vi "Match Terminals.vi"(10 "Terms[]":refnum<vi>[](array[refnum]), 11 "Terminals":T1[](array[typedef])) -> (3 "Terminals Out":T1[](array[typedef]))   [LabVIEW 2025]
uses:
  Controls/Terminal.ctl
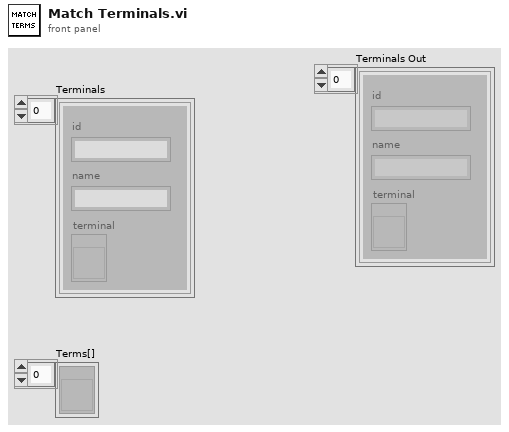
[diagram p1: front panel]
types:
  T1 = typedef "Terminal.ctl" = cluster{"id":string, "name":string, "terminal":refnum<vi>}
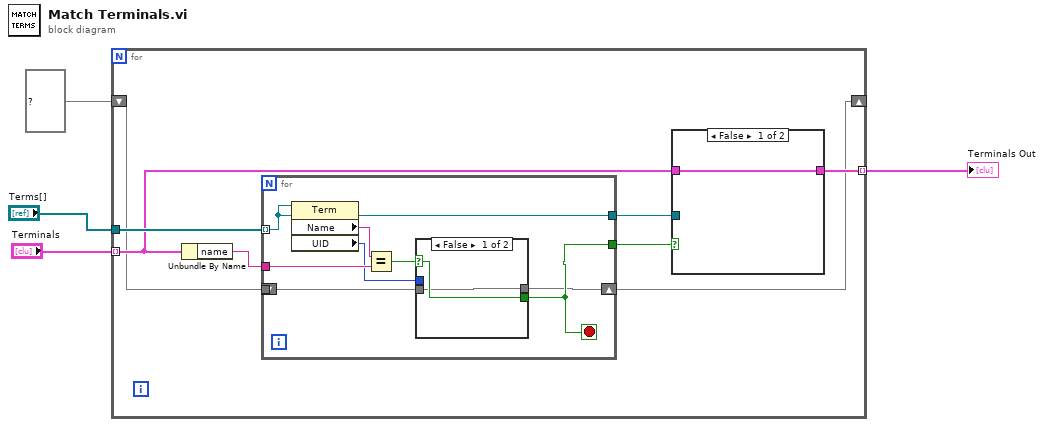
[diagram p0: block diagram]
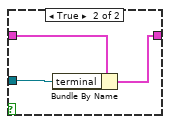
[diagram p2: hidden frame]
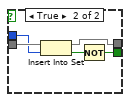
[diagram p3: hidden frame]
diagram:
  n1 = for {
    tunnel: "Terminals" -> [w9] mode=indexing
    tunnel: "Terms[]" -> [w12]
    tunnel: [w7] -> w2 mode=indexing
    shift-right: [w5] -> _
    shift-left: set{i32} {} ("set in") -> [w6]
    n2 = Unbundle By Name(w9) -> ("name"=w11:string)
    n3 = for {
      tunnel: w12 -> [w22] mode=indexing
      tunnel: w11 -> [w23]
      tunnel: [w18] -> w10
      tunnel: [w22] -> w8
      tunnel: w6 -> [w21]
      shift-right: [w17] -> w5
      shift-left: _ -> [_]
      stop <- w18 stop-if-true
      n4 = property class="Term"(reference=w22) -> ("Name"=w24:string, "UID"=w19:i32)  [unwired: 1 in, 2 out]
      n5 = Equal?(x=w24, y=w23) -> (x = y?=w20:bool)
      n6 = case shown="False" w20 {
        selector: w20 -> [w26 _]
        tunnel: w21 -> [w25 w31]
        tunnel: w19 -> [_ w30]
        tunnel: [w26 w28] -> w18
        tunnel: [w25 w27] -> w17
        frame False {
        }
        frame True {
          n7 = Insert Into Set(10:w30, 11:w31) -> (2:w29:bool, 3:w27:set{i32})
          n8 = Not(x=w29) -> (.not. x?=w28:bool)
        }
      }
    }
    n9 = case shown="False" w10 {
      tunnel: w9 -> [w13 w15]
      tunnel: w8 -> [_ w16]
      tunnel: [w13 w14] -> w7
      frame False {
      }
      frame True {
        n10 = Bundle By Name(cluster=w15, "terminal"=w16) -> (w14:T1)
      }
    }
  }
  "Terminals Out" <- w2
